vi "Reset Force Calibration Arrays.vi"(11 "array results in":T1) -> (3 "array results out":T1)   [LabVIEW 2020]
uses:
  Controller Loop/Controller Data.ctl
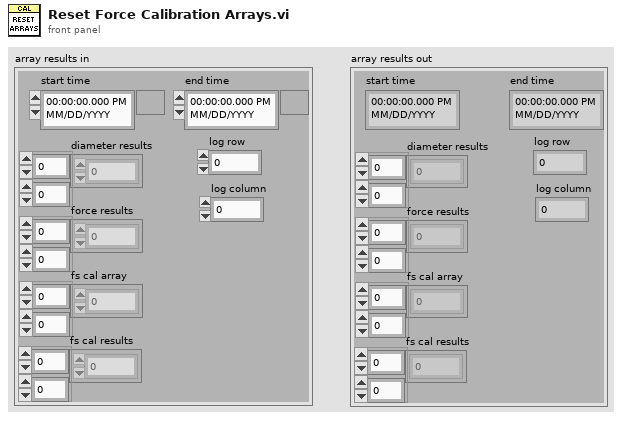
[diagram p1: front panel]
types:
  T1 = typedef "Controller Data.ctl" = cluster{"diameter results":dbl[][], "force results":dbl[][], "fs cal array":dbl[][], "fs cal results":dbl[][], "start time":timestamp, "end time":timestamp, "log row":i32, "log column":i32}
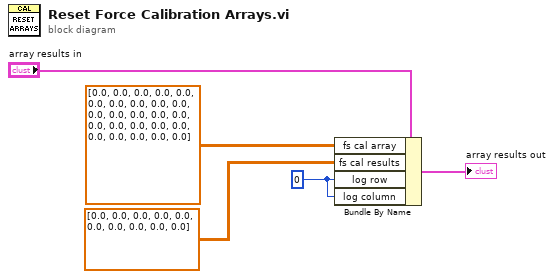
[diagram p0: block diagram]
diagram:
  w5 = u32 0 ("log number")
  n1 = Bundle By Name(cluster="array results in", "fs cal array"=dbl[][] [[0.0, 0.0, 0.0, 0.0, 0.0], [0.0, 0.0, 0.0, 0.0, 0.0], [0.0, 0.0, 0.0, 0.0, 0.0], [0.0, 0.0, 0.0, 0.0, 0.0], [0.0, 0.0, 0.0, 0.0, 0.0]], "fs cal results"=dbl[][] [[0.0, 0.0, 0.0, 0.0, 0.0], [0.0, 0.0, 0.0, 0.0, 0.0]] ("fs cal array"), "log row"=w5, "log column"=w5) -> (→"array results out":T1)
